vi "Configure Existing Segments.vi"(7 "Action (0: Add)":i32(ring) items=["Add", "Delete"], 8 "error in (no error)":errorcluster, 9 "Segment Number (1)":i32=1, 10 "Channel (1)":i32=1, 11 "VISA resource name":refnum<visa-resource-name>) -> (0 "error out":errorcluster, 3 "VISA resource name out":refnum<visa-resource-name>)   [LabVIEW 2018, in "Keysight PNA Series.lvlib"]
doc: "Adds or deletes a segment."
uses:
  Keysight PNA Series.lvlib
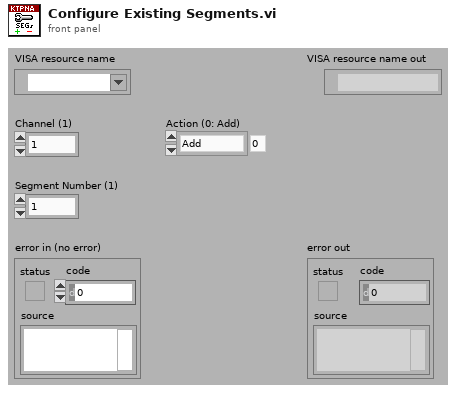
[diagram p1: front panel]
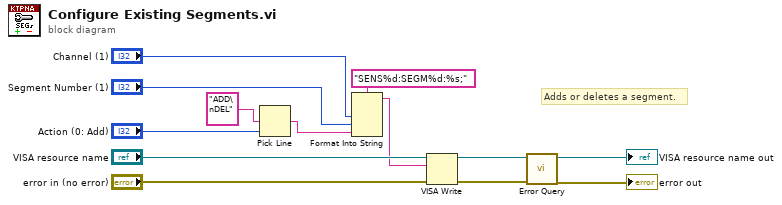
[diagram p0: block diagram]
diagram:
  # "Adds or deletes a segment."
  n1 = Pick Line(multi-line string="ADD\nDEL", line index="Action (0: Add)") -> (output string=w8:string)  [unwired: 1 in]
  n2 = Format Into String(format string="SENS%d:SEGM%d:%s;", "Channel (1)", "Segment Number (1)", w8) -> (resulting string=w1:string)  [unwired: 2 in, 1 out]
  n3 = VISA Write(VISA resource name="VISA resource name", write buffer=w1, error in (no error)="error in (no error)") -> (VISA resource name out=w5:refnum<visa-resource-name>, error out=w4:errorcluster)  [unwired: 1 out]
  n4 = call "Error Query.vi"("error in (no error)"=w4, "VISA resource name"=w5) -> ("error out"=→"error out":errorcluster, "VISA resource name out"=→"VISA resource name out":refnum<visa-resource-name>)  [unwired: 6 in, 2 out]
